vi "Release Server Message Queues.vi"(8 "error in (no error)":errorcluster, 11 "Server Message Queues":T1) -> (0 "error out":errorcluster)   [LabVIEW 2024, in "Message Queue.lvlib"]
doc: "Releases the message queues of the server."
uses:
  Message Queue.lvlib
  Server Message Queues.ctl
  Message Cluster.ctl
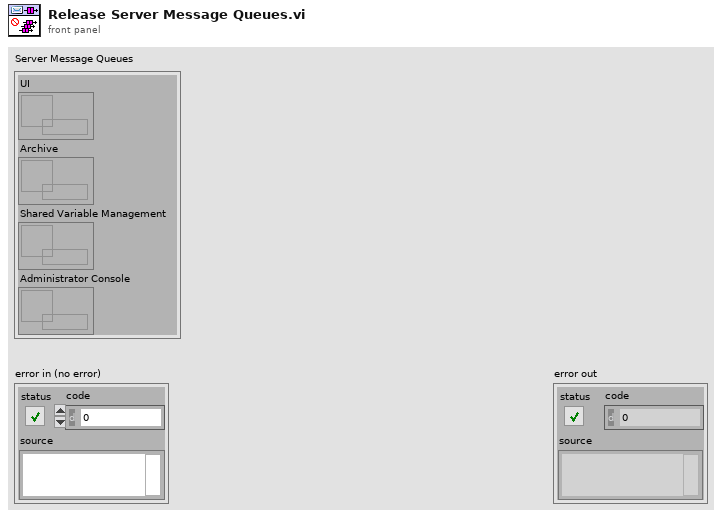
[diagram p1: front panel]
types:
  T1 = typedef "Message Queue.lvlib/Server Message Queues.ctl" = cluster{"UI":refnum<queue>, "Archive":refnum<queue>, "Shared Variable Management":refnum<queue>, "Administrator Console":refnum<queue>}
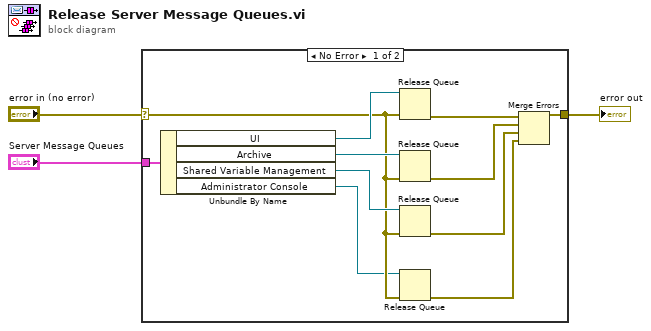
[diagram p0: block diagram]
diagram:
  n1 = case shown="No Error" "error in (no error)" {
    selector: "error in (no error)" -> [w6 w15]
    tunnel: [w8 w15] -> w3
    tunnel: "Server Message Queues" -> [w7 _]
    frame No Error {
      n2 = Unbundle By Name(w7) -> ("UI"=w9:refnum<queue>, "Archive"=w10:refnum<queue>, "Shared Variable Management"=w11:refnum<queue>, "Administrator Console"=w4:refnum<queue>)
      n3 = Release Queue(queue=w9, error in (no error)=w6) -> (error out=w12:errorcluster)  [unwired: 1 in, 2 out]
      n4 = Release Queue(queue=w10, error in (no error)=w6) -> (error out=w13:errorcluster)  [unwired: 1 in, 2 out]
      n5 = Release Queue(queue=w11, error in (no error)=w6) -> (error out=w14:errorcluster)  [unwired: 1 in, 2 out]
      n6 = Release Queue(queue=w4, error in (no error)=w6) -> (error out=w5:errorcluster)  [unwired: 1 in, 2 out]
      n7 = Merge Errors(w12, w13, w14, w5) -> (w8:errorcluster)
    }
    frame Error {
    }
  }
  "error out" <- w3
